vi "ChkDateTime.vi"(11 "文字列":string) -> (3 "ブール":bool)   [LabVIEW 2014]
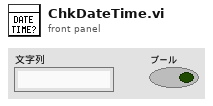
[diagram p1: front panel]
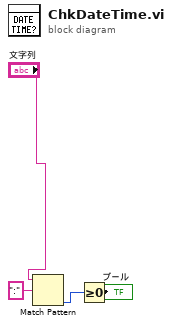
[diagram p0: block diagram]
diagram:
  n1 = Match Pattern(string="文字列", regular expression=":" ("正規表現")) -> (offset past match=w2:i32)  [unwired: 1 in, 3 out]
  n2 = Greater Or Equal To 0?(x=w2) -> (x >= 0?=→"ブール":bool)
